vi "Constructor.vi"(8 "error in":errorcluster, 9 "Value":string, 10 "Name":string, 11 "String in":refnum<class "String.lvclass">) -> (0 "error out":errorcluster, 3 "String out":refnum<class "String.lvclass">)   [LabVIEW 2021, in "ProligentXMLGenerator.lvlib" / "String.lvclass"]
uses:
  String.lvclass
  String.lvclass/String.ctl
  Attribute/Attribute.lvclass
  C:/Projects/proligent-xml-generator-labview/src/ProligentXMLGenerator/Base/Attribute/Attribute.lvclass
  C:/Projects/proligent-xml-generator-labview/src/ProligentXMLGenerator/Base/String/String.lvclass
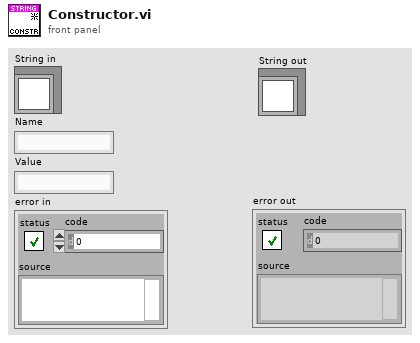
[diagram p1: front panel]
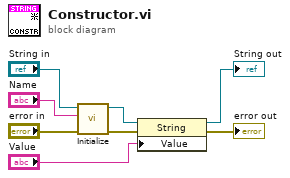
[diagram p0: block diagram]
diagram:
  n1 = call "Initialize.vi"("error in"="error in", "Name"="Name", "Attribute in"="String in") -> ("error out"=w3:errorcluster, "Attribute out"=w4:refnum<class "String.lvclass">)  [unwired: 7 in]
  n2 = property on="Property Node" class="String"(reference=w4, error in=w3, "Value"="Value") -> (reference out=→"String out":refnum<class "String.lvclass">, error out=→"error out":errorcluster)
